vi "CRYFlatten Data.vi"(11 "Datum":T1={"Name"="", "Curve"=[], "X data"=1, "Y data"=1, "Z data"=1, "X axis"=0, "Y axis"=1, "Z axis"=1, "X unit"="", "Y unit"="", "Z unit"="", "X dB ref"=1.0, "Y dB ref"=1.0, "Z dB ref"=1.0, "single val"=FALSE, "protected"=FALSE, "display X"=TRUE, "display Y"=FALSE, "display Z"=TRUE, "Test Info"="", "Step No."=0, "Plot Settings"={"Color"=0, "Interpolation"=0, "Point Style"=0, "Line Style"=0, "Point Color"=0, "Line Width"=0, "Bar Plot Style"=0, "Fill To"=0}, "AutoProtect"=FALSE} {"Z data" items=["dB", "Lin"]; "X data" items=["dB", "Lin"]; "Y data" items=["dB", "Lin"]; "Z dB ref" format="%.1f"; "Z axis" items=["Log", "Lin"]; "X dB ref" format="%.1f"; "X axis" items=["Log", "Lin"]; "Y axis" items=["Log", "Lin"]; "Y dB ref" format="%.1f"; "Curve"."z" format="%.2f"; "Curve"."y" format="%.2f"; "Curve"."x" format="%.2f"}) -> (3 "Data flattened":string)   [LabVIEW 2013]
uses:
  Typedef Control/CRYData Cluster.ctl
  Typedef Control/CRYData Cluster SC.ctl
  Typedef Control/CRYAxis Unit Type.ctl
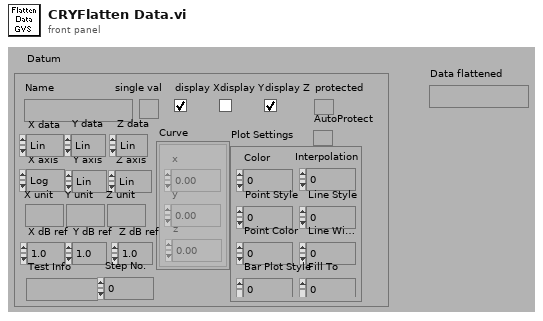
[diagram p1: front panel]
types:
  T1 = typedef "CRYData Cluster.ctl" = cluster{"Name":string, "Curve":cluster{"x":dbl, "y":dbl, "z":dbl}[], "X data":u16, "Y data":u16, "Z data":u16, "X axis":u16, "Y axis":u16, "Z axis":u16, "X unit":string, "Y unit":string, "Z unit":string, "X dB ref":dbl, "Y dB ref":dbl, "Z dB ref":dbl, "single val":bool, "protected":bool, "display X":bool, "display Y":bool, "display Z":bool, "Test Info":string, "Step No.":i32, "Plot Settings":cluster{"Color":u32, "Interpolation":u8, "Point Style":u8, "Line Style":u8, "Point Color":u32, "Line Width":u8, "Bar Plot Style":u8, "Fill To":i16}, "AutoProtect":bool}
  T2 = typedef "CRYData Cluster SC.ctl" = cluster{"Name":string, "Curve":cluster{"x":dbl, "y":dbl, "z":dbl}[], "X data":T3, "Y data":T3, "Z data":T3, "X axis":u16, "Y axis":u16, "Z axis":u16, "X unit":string, "Y unit":string, "Z unit":string, "X dB ref":dbl, "Y dB ref":dbl, "Z dB ref":dbl, "single val":bool, "protected":bool, "display X":bool, "display Y":bool, "display Z":bool, "Plot Settings":cluster{"Color":u32, "Interpolation":u8, "Point Style":u8, "Line Style":u8, "Point Color":u32, "Line Width":u8, "Bar Plot Style":u8, "Fill To":i16}, "Test Info":string}
  T3 = typedef "CRYAxis Unit Type.ctl" = u16
  T4 = cluster{"Color":u32, "Interpolation":u8, "Point Style":u8, "Line Style":u8, "Point Color":u32, "Line Width":u8, "Bar Plot Style":u8, "Fill To":i16}
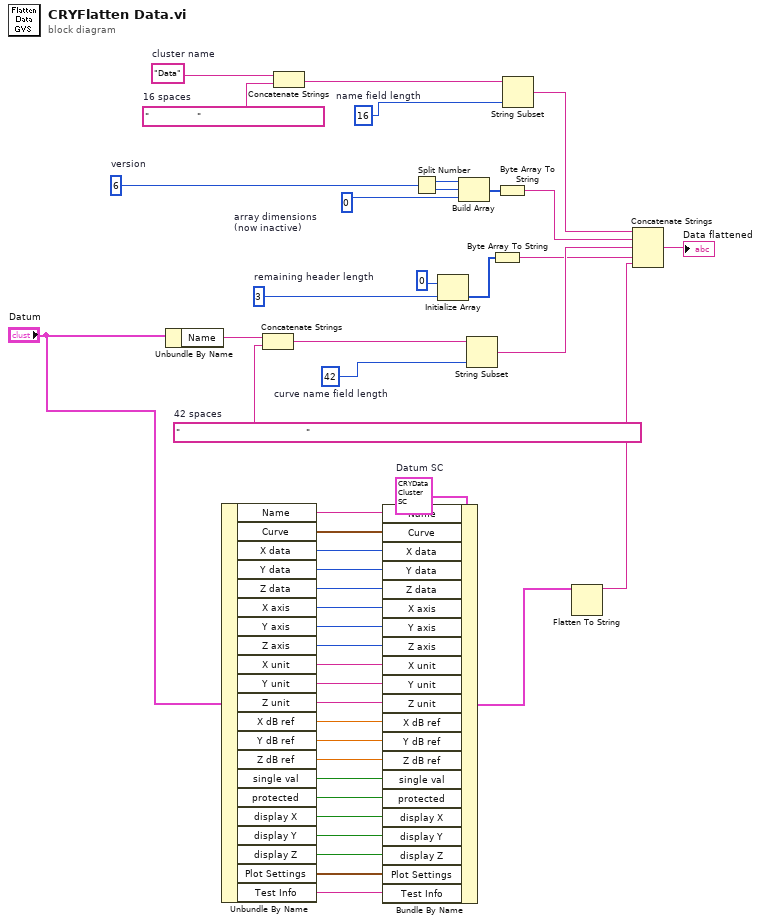
[diagram p0: block diagram]
diagram:
  w25 = u16 6  # version
  w24 = T2 {"Name"="", "Curve"=[], "X data"=1, "Y data"=1, "Z data"=1, "X axis"=0, "Y axis"=1, "Z axis"=1, "X unit"="Hz", "Y unit"="", "Z unit"="deg.", "X dB ref"=1.0, "Y dB ref"=1.0, "Z dB ref"=1.0, "single val"=FALSE, "protected"=FALSE, "display X"=TRUE, "display Y"=TRUE, "display Z"=TRUE, "Plot Settings"={"Color"=0, "Interpolation"=2, "Point Style"=0, "Line Style"=0, "Point Color"=0, "Line Width"=0, "Bar Plot Style"=0, "Fill To"=-1}, "Test Info"=""}  # Datum SC
  w28 = 3  # remaining header length
  w36 = 42  # curve name field length
  w34 = "                                          "  # 42 spaces
  w38 = u8 0  # array dimensions (now inactive)
  w40 = 16  # name field length
  w41 = "                "  # 16 spaces
  w42 = "Data"  # cluster name
  n1 = Unbundle By Name("Datum") -> ("Name"=w35:string)
  n2 = Unbundle By Name("Datum") -> ("Name"=w22:string, "Curve"=w21:cluster{"x":dbl, "y":dbl, "z":dbl}[], "X data"=w20:u16, "Y data"=w19:u16, "Z data"=w18:u16, "X axis"=w17:u16, "Y axis"=w16:u16, "Z axis"=w15:u16, "X unit"=w14:string, "Y unit"=w13:string, "Z unit"=w12:string, "X dB ref"=w11:dbl, "Y dB ref"=w10:dbl, "Z dB ref"=w9:dbl, "single val"=w8:bool, "protected"=w7:bool, "display X"=w6:bool, "display Y"=w5:bool, "display Z"=w4:bool, "Plot Settings"=w3:T4, "Test Info"=w2:string)
  n3 = Concatenate Strings(w35, w34) -> (w37:string)
  n4 = Concatenate Strings(w42, w41) -> (w39:string)
  n5 = Bundle By Name(cluster=w24, "Name"=w22, "Curve"=w21, "X data"=w20, "Y data"=w19, "Z data"=w18, "X axis"=w17, "Y axis"=w16, "Z axis"=w15, "X unit"=w14, "Y unit"=w13, "Z unit"=w12, "X dB ref"=w11, "Y dB ref"=w10, "Z dB ref"=w9, "single val"=w8, "protected"=w7, "display X"=w6, "display Y"=w5, "display Z"=w4, "Plot Settings"=w3, "Test Info"=w2) -> (w23:T2)
  n6 = Split Number(x=w25) -> (hi(x)=w46:u8, lo(x)=w45:u8)
  n7 = Initialize Array(u8 0, w28) -> (w27:u8[])
  n8 = Build Array(w46, w45, w38) -> (w44:u8[])
  n9 = String Subset(string=w37, length (rest)=w36) -> (substring=w31:string)  [unwired: 1 out]
  n10 = Byte Array To String(unsigned byte array=w27) -> (string=w26:string)
  n11 = Byte Array To String(unsigned byte array=w44) -> (string=w32:string)
  n12 = String Subset(string=w39, length (rest)=w40) -> (substring=w33:string)  [unwired: 1 out]
  n13 = Flatten To String(anything=w23) -> (data string=w30:string)  [unwired: 1 in, 4 out]
  n14 = Concatenate Strings(w33, w32, w31, w26, w30) -> (→"Data flattened":string)
